vi "AIT 664 - ReadWrite Channels.vi"(0 "Channels In":T1[](array[typedef]) {"Message Settings"."Transmit Channel Data Reference" format="%.0x"; "Message Settings"."Queue Transmit Channel" format="%.0x"; "Message Settings"."Driver Data"."Num Bits" min=1 max=32; "Message Settings"."Block Data Refs"."Data Reference" format="%.0x"; "Rx Com Udp Port"."Handle" format="%08x"; "Tx Com Udp Port"."Handle" format="%08x"}, 1 "Mode":T13, 5 "FIFOs In":T14, 7 "Channel Index":i32, 11 "error in (no error)":errorcluster, 12 "Iteration":i32) -> (4 "Channels Out":T1[](array[typedef]) {"Message Settings"."Transmit Channel Data Reference" format="%.0x"; "Message Settings"."Queue Transmit Channel" format="%.0x"; "Message Settings"."Driver Data"."Num Bits" min=1 max=32; "Message Settings"."Block Data Refs"."Data Reference" format="%.0x"; "Rx Com Udp Port"."Handle" format="%08x"; "Tx Com Udp Port"."Handle" format="%08x"}, 6 "FIFOs Out":T14, 15 "error out":errorcluster)   [LabVIEW 2013, in "AIT 664 Custom Device.lvlib"]
doc: "Move data between the hardware / RT and RT / Veristand."
uses:
  AIT 664 Custom Device.lvlib
  RT Controls/FIFO.ctl
  RT Controls/ReadWrite Selector.ctl
  RT Controls/AIT 664 - RT Hardware Channel.ctl
  RT Controls/AIT 664 - RT Message Settings.ctl
  <vilib>/NI Veristand/Custom Device API/Block Data Reference.ctl
  <vilib>/NI Veristand/Custom Device API/Data Reference.ctl
  RT Controls/AIT 664 - Driver Data.ctl
  Controls and Global/Start Bit.ctl
  Controls and Global/Number of Bits.ctl
  <vilib>/NI Veristand/Custom Device API/Custom Device Item Ref.ctl
  <userlib>/ARINC 664/AIT 664 Controls/General/Message Port.ctl
  <userlib>/ARINC 664/AIT 664 Controls/General/Direction.ctl
  <userlib>/ARINC 664/AIT 664 Controls/General/Message Port Type.ctl
  System Explorer/Controls/664 - Sampling Type.ctl
  <instrlib>/AIT 664/Public/Action-Status/Rx/AIT 664 Rx Get Message Port Status.vi
  <instrlib>/AIT 664/Public/Data/Rx/AIT 664 Rx Read.vi
  <instrlib>/AIT 664/Private/AIT 664 Data/Rx/Read/AIT 664 Rx Read (ComUdp).vi
  <vilib>/NI Veristand/Custom Device Tools/Custom Device Utility Library/NI VeriStand - Print Debug String.vi
  <vilib>/NI Veristand/Custom Device API/Custom Device API.lvlib
  <userlib>/ARINC 664/AIT 664 API.lvlib
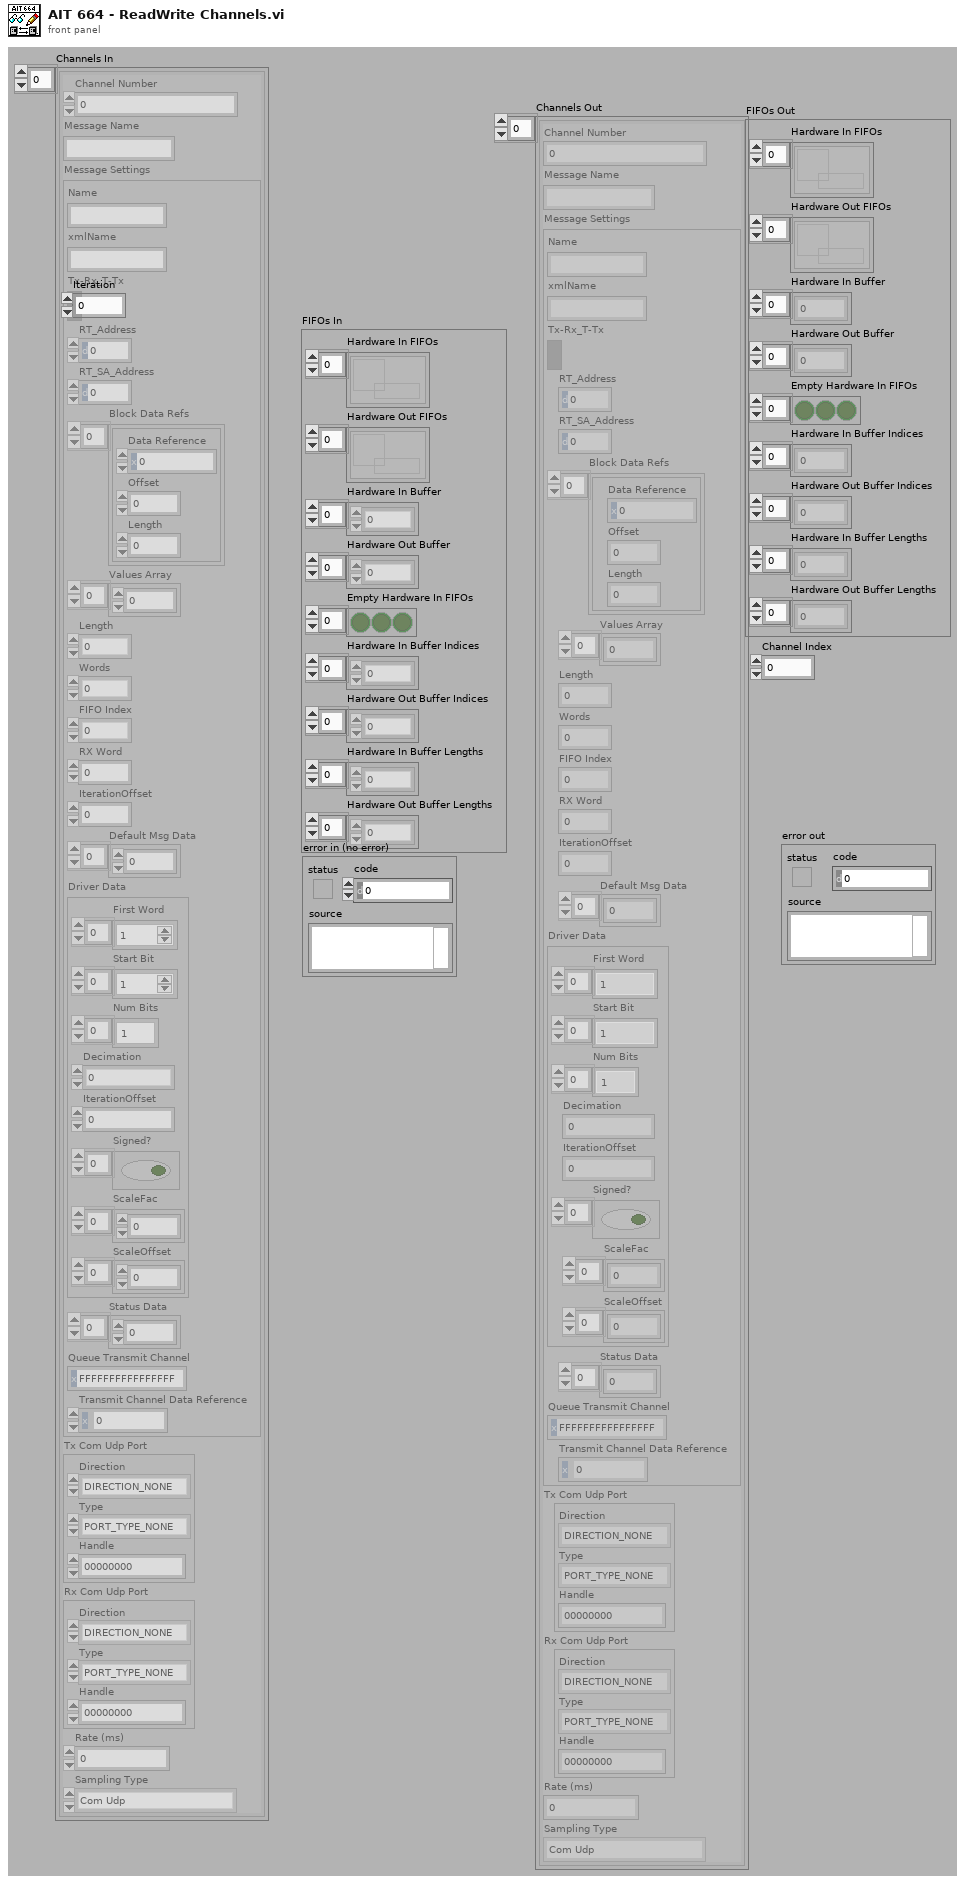
[diagram p1: front panel]
types:
  T1 = typedef "AIT 664 Custom Device.lvlib/AIT 664 - RT Hardware Channel.ctl" = cluster{"Channel Number":u16, "Message Name":string, "Message Settings":T2, "Tx Com Udp Port":T9, "Rx Com Udp Port":T9, "Rate (ms)":u32, "Sampling Type":T12}
  T2 = typedef "AIT 664 Custom Device.lvlib/AIT 664 - RT Message Settings.ctl" = cluster{"Name":string, "xmlName":string, "Tx-Rx_T-Tx":bool, "RT_Address":u8, "RT_SA_Address":u8, "Block Data Refs":T3[], "Values Array":dbl[], "Length":i32, "Words":i32, "FIFO Index":i32, "RX Word":u32, "IterationOffset":i32, "Default Msg Data":u8[], "Driver Data":T5, "Status Data":u32[], "Queue Transmit Channel":T8, "Transmit Channel Data Reference":T4}
  T3 = typedef "Custom Device API.lvlib/Block Data Reference.ctl" = cluster{"Data Reference":T4, "Offset":i32, "Length":i32}
  T4 = typedef "Custom Device API.lvlib/Data Reference.ctl" = i32
  T5 = typedef "AIT 664 Custom Device.lvlib/AIT 664 - Driver Data.ctl" = cluster{"First Word":T6[], "Start Bit":T6[], "Num Bits":T7[], "Decimation":i32, "IterationOffset":i32, "Signed?":bool[], "ScaleFac":dbl[], "ScaleOffset":dbl[]}
  T6 = typedef "AIT 664 Custom Device.lvlib/Start Bit.ctl" = i32
  T7 = typedef "AIT 664 Custom Device.lvlib/Number of Bits.ctl" = i32
  T8 = typedef "Custom Device API.lvlib/Custom Device Item Ref.ctl" = u64
  T9 = typedef "AIT 664 API.lvlib/Message Port.ctl" = cluster{"Direction":T10, "Type":T11, "Handle":u64}
  T10 = typedef "AIT 664 API.lvlib/Direction.ctl" = enum16{"DIRECTION_NONE", "DIRECTION_TX", "DIRECTION_RX"}
  T11 = typedef "AIT 664 API.lvlib/Message Port Type.ctl" = enum16{"PORT_TYPE_NONE", "COM_UDP", "SAP_UDP", "SAP_IP", "SAP_MAC", "COTS_MAC", "COTS_MAC_RAW"}
  T12 = typedef "AIT 664 Custom Device.lvlib/664 - Sampling Type.ctl" = enum16{"Com Udp", "Com Udp Queuing", "Sap Udp", "Sap Ip", "Sap Mac", "Unknown"}
  T13 = typedef "AIT 664 Custom Device.lvlib/ReadWrite Selector.ctl" = enum16{"Inline Read", "Inline Write", "Async HWIn", "Async HWOut"}
  T14 = typedef "AIT 664 Custom Device.lvlib/FIFO.ctl" = cluster{"Hardware In FIFOs":refnum<k33>[], "Hardware Out FIFOs":refnum<k33>[], "Hardware In Buffer":dbl[], "Hardware Out Buffer":dbl[], "Empty Hardware In FIFOs":bool[], "Hardware In Buffer Indices":i32[], "Hardware Out Buffer Indices":i32[], "Hardware In Buffer Lengths":i32[], "Hardware Out Buffer Lengths":i32[]}
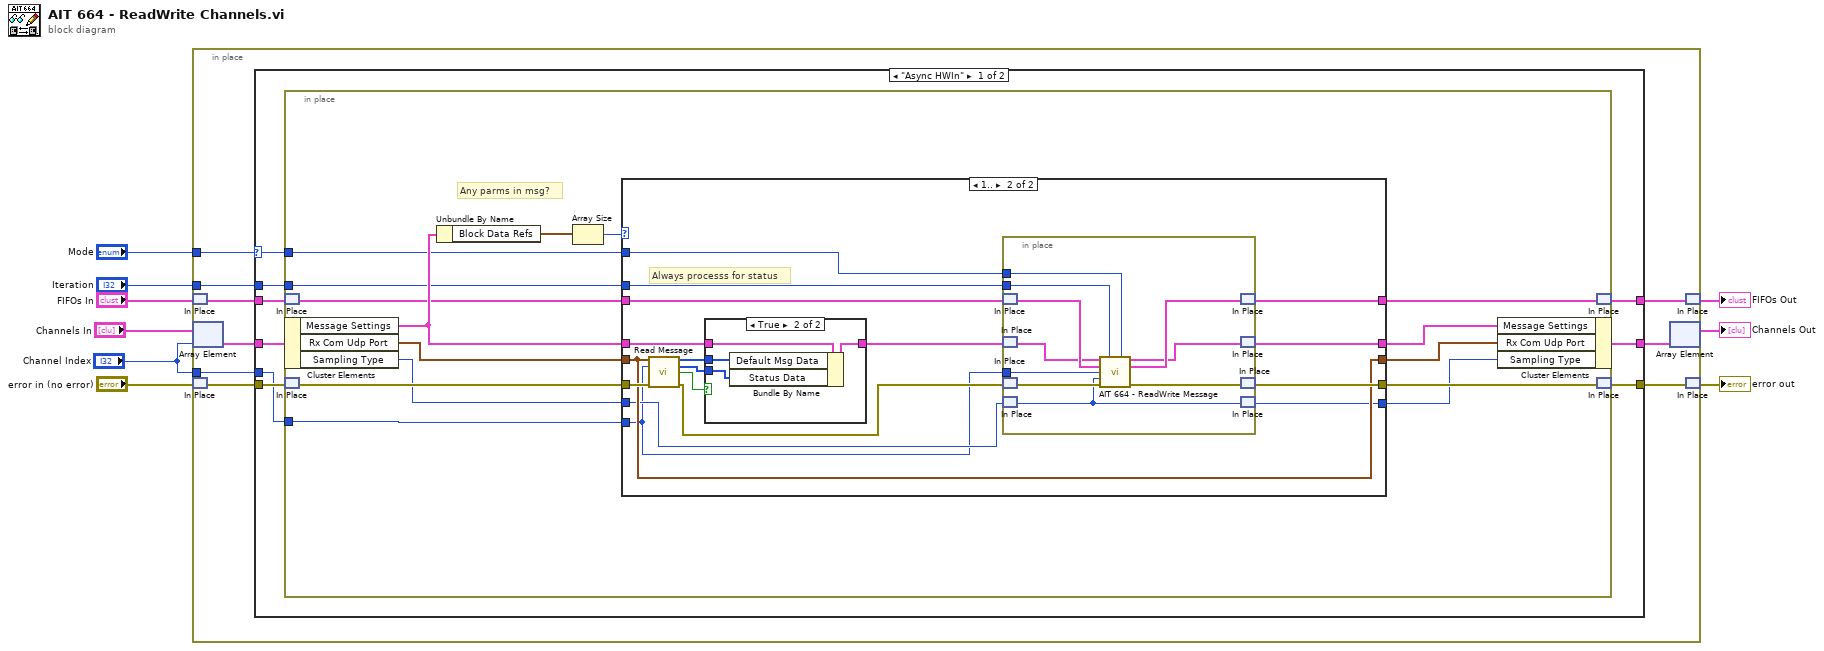
[diagram p0: block diagram]
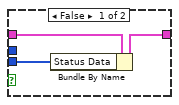
[diagram p3: hidden frame]
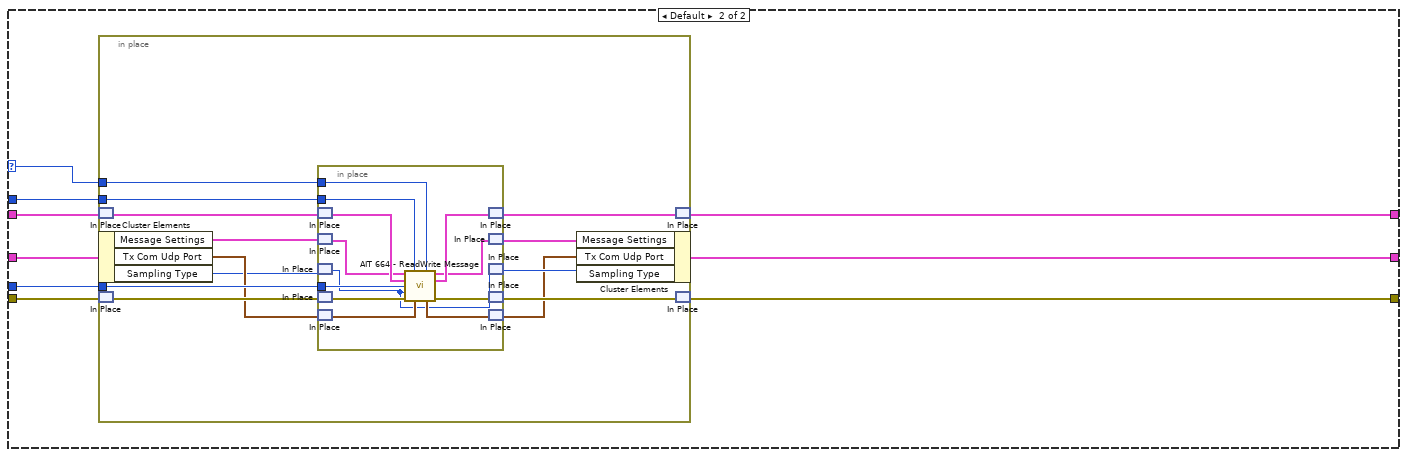
[diagram p4: hidden frame]
diagram:
  n1 = in-place {
    in-place-border: "Mode" -> [w12]
    in-place-border: "Iteration" -> [w13]
    in-place-border: "Channel Index" -> [w11]
    n2 = in-place-match #1("FIFOs In") -> (w15:T14)
    n3 = in-place-array #2("Channels In", "Channel Index") -> (w10:T1)
    n4 = in-place-match #3("error in (no error)") -> (w17:errorcluster)
    n5 = case shown="\"Async HWIn\"" w12 {
      selector: w12 -> [w21 w83]
      tunnel: w10 -> [w19 w90]
      tunnel: [w27 w89] -> w18
      tunnel: w17 -> [w26 w88]
      tunnel: [w25 w87] -> w16
      tunnel: w15 -> [w24 w86]
      tunnel: [w23 w85] -> w14
      tunnel: w13 -> [w22 w84]
      tunnel: w11 -> [w20 w82]
      frame "Async HWIn" {
        n6 = in-place {
          in-place-border: w21 -> [w39]
          in-place-border: w22 -> [w37]
          in-place-border: w20 -> [w35]
          # "Any parms in msg?"
          n7 = in-place-match #4(w24) -> (w36:T14)
          n8 = in-place-cluster #5(w19) -> ("Message Settings"=w42:T2, "Rx Com Udp Port"=w31:T9, "Sampling Type"=w29:T12)
          n9 = in-place-match #6(w26) -> (w30:errorcluster)
          n10 = Unbundle By Name(w42) -> ("Block Data Refs"=w33:T3[])
          n11 = Array Size(array=w33) -> (size(s)=w32:i32)
          n12 = case shown="1.." w32 {
            tunnel: w42 -> [w46 w58]
            tunnel: [w46 w64] -> w41
            tunnel: [w45 w63] -> w40
            tunnel: w39 -> [_ w62]
            tunnel: [w47 w61] -> w38
            tunnel: w37 -> [_ w60]
            tunnel: w36 -> [w47 w59]
            tunnel: w30 -> [w45 w55]
            tunnel: w35 -> [_ w48]
            tunnel: w31 -> [w44 w51]
            tunnel: [w44 w51] -> w34
            tunnel: w29 -> [w43 w49]
            tunnel: [w43 w50] -> w28
            frame 0, Default {
            }
            frame 1.. {
              # "Always processs for status"
              n13 = call "Read Message.vi"("Rx Com Udp Port"=w51, "Channel Index"=w48, "error in (no error)"=w55) -> ("data buffer out"=w52:u8[], "status data out"=w53:u32[], "Data Available"=w54:bool, "error out"=w56:errorcluster)  [unwired: 9 in]
              n14 = case shown="True" w54 {
                tunnel: w58 -> [w77 w81]
                tunnel: [w76 w80] -> w57
                tunnel: w52 -> [_ w79]
                tunnel: w53 -> [w75 w78]
                frame False {
                  n15 = Bundle By Name(cluster=w77, "Status Data"=w75) -> (w76:T2)
                }
                frame True {
                  n16 = Bundle By Name(cluster=w81, "Default Msg Data"=w79, "Status Data"=w78) -> (w80:T2)
                }
              }
              n17 = in-place {
                in-place-border: w62 -> [w72]
                in-place-border: w60 -> [w71]
                in-place-border: w48 -> [w65]
                n18 = in-place-match #7(w59) -> (w70:T14)
                n19 = in-place-match #8(w57) -> (w68:T2)
                n20 = in-place-match #9(w56) -> (w74:errorcluster)
                n21 = in-place-match #10(w49) -> (w66:T12)
                n22 = call "AIT 664 - ReadWrite Message.vi"("Message In"=w68, "Iteration"=w71, "Mode"=w72, "FIFOs In"=w70, "Channel Index"=w65, "Sampling Type"=w66, "error in (no error)"=w74) -> ("Message Out"=w67:T2, "FIFOs Out"=w69:T14, "error out"=w73:errorcluster)  [unwired: 5 in, 1 out]
                n23 = in-place-match #7(w69) -> (w61:T14)
                n24 = in-place-match #8(w67) -> (w64:T2)
                n25 = in-place-match #9(w73) -> (w63:errorcluster)
                n26 = in-place-match #10(w66) -> (w50:T12)
              }
            }
          }
          n27 = in-place-cluster #5("Message Settings"=w41, "Rx Com Udp Port"=w34, "Sampling Type"=w28) -> (w27:T1)
          n28 = in-place-match #4(w38) -> (w23:T14)
          n29 = in-place-match #6(w40) -> (w25:errorcluster)
        }
      }
      frame Default {
        n30 = in-place {
          in-place-border: w83 -> [w102]
          in-place-border: w84 -> [w100]
          in-place-border: w82 -> [w97]
          n31 = in-place-match #11(w86) -> (w99:T14)
          n32 = in-place-cluster #12(w90) -> ("Message Settings"=w95:T2, "Tx Com Udp Port"=w96:T9, "Sampling Type"=w93:T12)
          n33 = in-place-match #13(w88) -> (w98:errorcluster)
          n34 = in-place {
            in-place-border: w102 -> [w113]
            in-place-border: w100 -> [w114]
            in-place-border: w97 -> [w109]
            n35 = in-place-match #14(w99) -> (w110:T14)
            n36 = in-place-match #15(w95) -> (w106:T2)
            n37 = in-place-match #16(w93) -> (w104:T12)
            n38 = in-place-match #17(w98) -> (w111:errorcluster)
            n39 = in-place-match #18(w96) -> (w108:T9)
            n40 = call "AIT 664 - ReadWrite Message.vi"("Message In"=w106, "Iteration"=w114, "Mode"=w113, "FIFOs In"=w110, "Channel Index"=w109, "Sampling Type"=w104, "error in (no error)"=w111, "Tx Com Udp Port"=w108) -> ("Message Out"=w105:T2, "FIFOs Out"=w112:T14, "Tx Com Udp Port out"=w107:T9, "error out"=w115:errorcluster)  [unwired: 4 in]
            n41 = in-place-match #14(w112) -> (w101:T14)
            n42 = in-place-match #15(w105) -> (w94:T2)
            n43 = in-place-match #16(w104) -> (w92:T12)
            n44 = in-place-match #17(w115) -> (w103:errorcluster)
            n45 = in-place-match #18(w107) -> (w91:T9)
          }
          n46 = in-place-cluster #12("Message Settings"=w94, "Tx Com Udp Port"=w91, "Sampling Type"=w92) -> (w89:T1)
          n47 = in-place-match #11(w101) -> (w85:T14)
          n48 = in-place-match #13(w103) -> (w87:errorcluster)
        }
      }
    }
    n49 = in-place-array #2(w18) -> (→"Channels Out":T1[])  [unwired: 1 out]
    n50 = in-place-match #1(w14) -> (→"FIFOs Out":T14)
    n51 = in-place-match #3(w16) -> (→"error out":errorcluster)
  }
